vi "Send initialize.vi"(7 "Message Priority (Normal)":T1=enum."Normal", 8 "error in (no error)":errorcluster, 10 "file path (use dialog)":path, 11 "Message Enqueuer":refnum<class "Message Enqueuer.lvclass">) -> (0 "error out":errorcluster, 3 "Message Enqueuer out":refnum<class "Message Enqueuer.lvclass">)   [LabVIEW 2017, in "Data Logger.lvlib" / "initialize Msg.lvclass"]
doc: "This VI sends the message to an actor."
uses:
  initialize Msg.lvclass
  <vilib>/ActorFramework/Message Enqueuer/Message Enqueuer.lvclass
  <vilib>/ActorFramework/Message Enqueuer/Message Priority.ctl
  C:/Program Files (x86)/National Instruments/LabVIEW 2017/vi.lib/ActorFramework/Message/Message.lvclass
  initialize Msg.lvclass/initialize Msg.ctl
  <vilib>/ActorFramework/Message Enqueuer/Message Enqueuer.lvclass/Message Enqueuer.ctl
  <vilib>/ActorFramework/Message Priority Queue/Priority Enqueue.vi
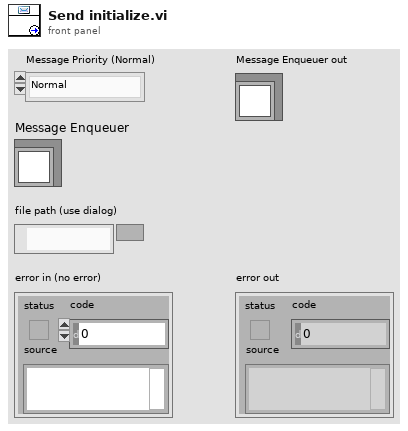
[diagram p1: front panel]
types:
  T1 = typedef "Actor Framework.lvlib/Message Enqueuer.lvclass/Message Priority.ctl" = enum16{"Low", "Normal", "High"}
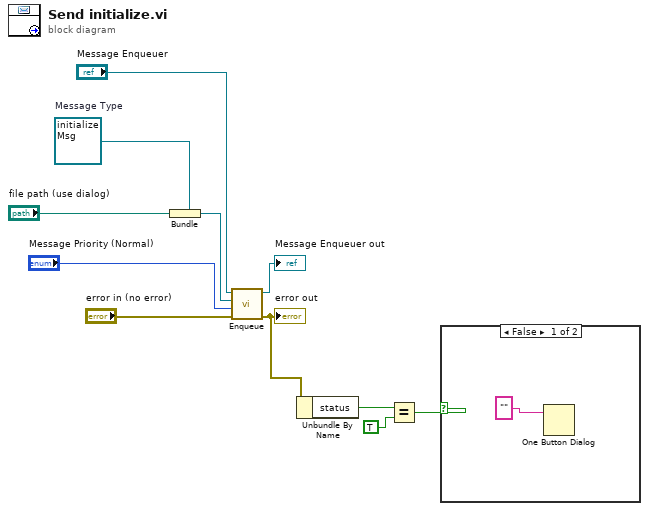
[diagram p0: block diagram]
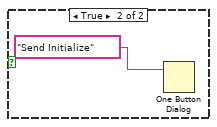
[diagram p2: hidden frame]
diagram:
  w6 = refnum<class "initialize Msg.lvclass"> refnum  # Message Type
  n1 = Bundle(cluster=w6, "file path (use dialog)") -> (w7:refnum<class "initialize Msg.lvclass">)
  n2 = call <vilib>:"Enqueue.vi"("error in (no error)"="error in (no error)", "Message Priority (Normal)"="Message Priority (Normal)", "Message"=w7, "Message Enqueuer in"="Message Enqueuer") -> ("error out"=w3:errorcluster, "Message Enqueuer out"=→"Message Enqueuer out":refnum<class "Message Enqueuer.lvclass">)  [unwired: 6 in]
  "error out" <- w3
  n3 = Unbundle By Name(w3) -> ("status"=w2:bool)
  n4 = Equal?(x=w2, y=TRUE) -> (x = y?=w1:bool)
  n5 = case shown="False" w1 {
    frame False {
      n6 = One Button Dialog(message="") -> ()  [unwired: 1 in, 1 out]
    }
    frame True {
      n7 = One Button Dialog(message="Send Initialize") -> ()  [unwired: 1 in, 1 out]
    }
  }
